vi "Write HDF5.vi"(8 "error in (no error)":errorcluster, 10 "path":path, 11 "LVtoITX in":refnum<class "LVtoITX.lvclass">) -> (0 "error out":errorcluster, 3 "LVtoITX out":refnum<class "LVtoITX.lvclass">)   [LabVIEW 2016]
uses:
  <vilib>/addons/h5labview2/file/H5Fmode.ctl
  <vilib>/addons/h5labview2/file/H5F.lvlib
  <vilib>/addons/h5labview2/base/hid_t.ctl
  <vilib>/addons/h5labview2/dataset/H5Dwrite.llb/H5Dwrite.xnode
  <vilib>/addons/h5labview2/base/H5Equery.vi
  <vilib>/addons/h5labview2/base/lib_path.vi
  LVtoITX.lvclass
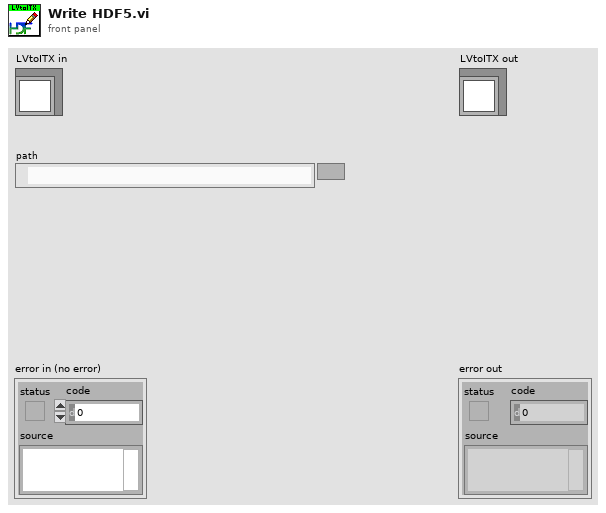
[diagram p1: front panel]
types:
  T1 = typedef "H5F.lvlib/H5Fmode.ctl" = enum16{"read-only", "read-write", "overwrite", "create new", "open or create"}
  T2 = typedef "hid_t.ctl" = i32
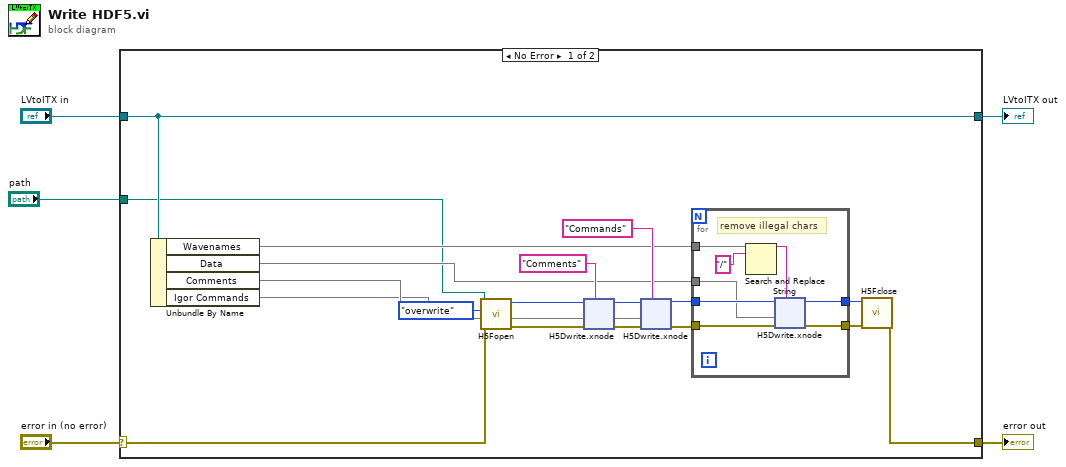
[diagram p0: block diagram]
diagram:
  n1 = case shown="No Error" "error in (no error)" {
    selector: "error in (no error)" -> [w7 w90]
    tunnel: [w17 w90] -> w2
    tunnel: [w16 w91] -> w3
    tunnel: "LVtoITX in" -> [w16 w91]
    tunnel: "path" -> [w6 _]
    frame No Error {
      n2 = Unbundle By Name(w16) -> ("Wavenames"=w15, "Data"=w14, "Comments"=w13, "Igor Commands"=w12)
      n3 = call <vilib>:"H5Fopen.vi"("error in (no error)"=w7, "mode (read-only)"=H5Fmode."overwrite" ("mode"), "path"=w6) -> ("error out"=w8:errorcluster, "ref out"=w10:T2)  [unwired: 7 in]
      n4 = xnode "H5Dwrite.xnode"("dataset name"="Comments" ("attrib name"), "error in (no error)"=w8, "data"=w13, "ref in"=w10) -> ("error out"=w22:errorcluster, "ref out"=w21:T2)  [unwired: 3 in, 1 out]
      n5 = xnode "H5Dwrite.xnode"("dataset name"="Commands" ("attrib name"), "error in (no error)"=w22, "data"=w12, "ref in"=w21) -> ("error out"=w20:errorcluster, "ref out"=w18:T2)  [unwired: 3 in, 1 out]
      n6 = for {
        tunnel: w15 -> [w66]
        tunnel: w14 -> [w63]
        tunnel: w18 -> [w68]
        tunnel: [w67] -> w9
        tunnel: w20 -> [w69]
        tunnel: [w70] -> w11
        # "remove illegal chars"
        n7 = Search and Replace String(input string=w66, search string="/") -> (result string=w65:string)  [unwired: 6 in, 3 out]
        n8 = xnode "H5Dwrite.xnode"("dataset name"=w65, "error in (no error)"=w69, "data"=w63, "ref in"=w68) -> ("error out"=w70:errorcluster, "ref out"=w67:T2)  [unwired: 3 in, 1 out]
      }
      n9 = call <vilib>:"H5Fclose.vi"("error in (no error)"=w11, "ref"=w9) -> ("error out"=w17:errorcluster)  [unwired: 9 in]
    }
    frame Error {
    }
  }
  "error out" <- w2
  "LVtoITX out" <- w3
